vi "SetReference2.vi"(0 "DeviceType":u32, 1 "DeviceInd":u32, 2 "CANInd":u32, 3 "RefType":T1 items=["REFTYPE_MODE"=0, "REFTYPE_FILTER"=1, "REFTYPE_ACR0"=2, "REFTYPE_AMR0"=6, "REFTYPE_kCANBAUD"=10, "REFTYPE_CANRX_EN"=13, "REFTYPE_UARTBAUD"=14, "REFTYPE_ALL"=15, "REFTYPE_BRS"=16], 4 "pData":u8[](array[numeric]), 5 "error in (no error)":errorcluster caption="错误输入（无错误）") -> (14 "Success":bool, 19 "error out":errorcluster caption="错误输出")   [LabVIEW 2011]
uses:
  VIs/ParamType.ctl
  data/ControlCAN.dll
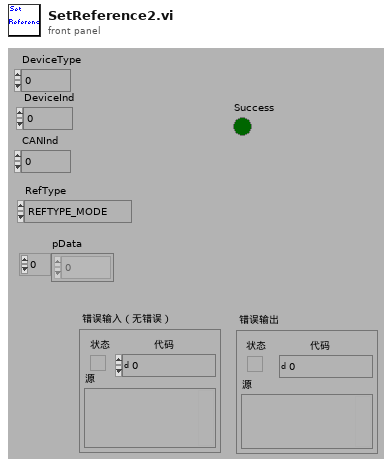
[diagram p1: front panel]
types:
  T1 = typedef "ParamType.ctl" = u32
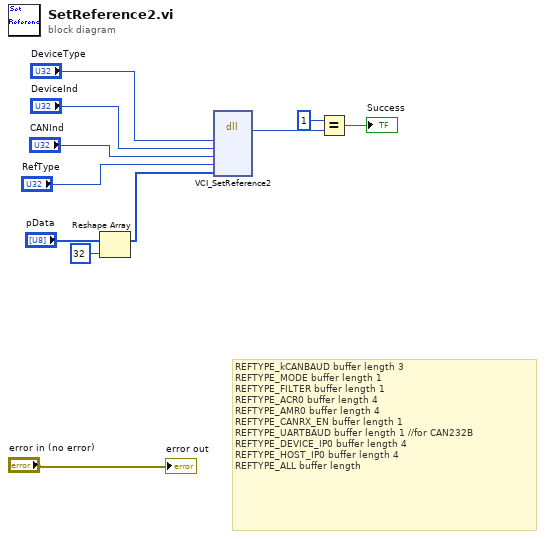
[diagram p0: block diagram]
diagram:
  # "REFTYPE_kCANBAUD buffer length 3\nREFTYPE_MODE buffer length 1\nREFTYPE_FILTER buffer length 1\nREFTYPE_ACR0 buffer length 4\nREFTYPE_AMR0 buffer length 4\nREFTYPE_CANRX_EN buffer length 1\nREFTYPE_UARTBAUD buffer length 1 //for CAN232B\nREFTYPE_DEVICE_IP0 buffer length 4\nREFTYPE_HOST_IP0 buffer length 4\nREFTYPE_ALL buffer length"
  n1 = Reshape Array("pData", 32 ("维数大小")) -> (w3:u8[])
  n2 = dll-call lib="PTH1Nabs D\t董海成\t上位机2.进行中USB-CAN TooldataControlCAN.dll" fn="VCI_SetReference2" label="VCI_SetReference"("DeviceType"="DeviceType", "DeviceInd"="DeviceInd", "CANInd"="CANInd", "RefType"="RefType", "pData"=w3) -> ("返回类型"=w7:u32)  [unwired: 8 in, 2 out]
  n3 = Equal?(x=u32 1, y=w7) -> (x = y?=→"Success":bool)
  "error out" <- "error in (no error)"
